vi "getAll.vi"(8 "error in (no error)":errorcluster, 11 "Instrument.sample-registry":refnum<class "Instrument.sample-registry.lvclass">) -> (0 "error out":errorcluster, 2 "getAll":variant, 3 "Instrument.sample-registry out":refnum<class "Instrument.sample-registry.lvclass">)   [LabVIEW 2019, in "Instrument.sample-registry.lvclass"]
uses:
  Instrument.sample-registry.lvclass
  Typedefs/Instrument.sample-registry.getAll--Cluster.ctl
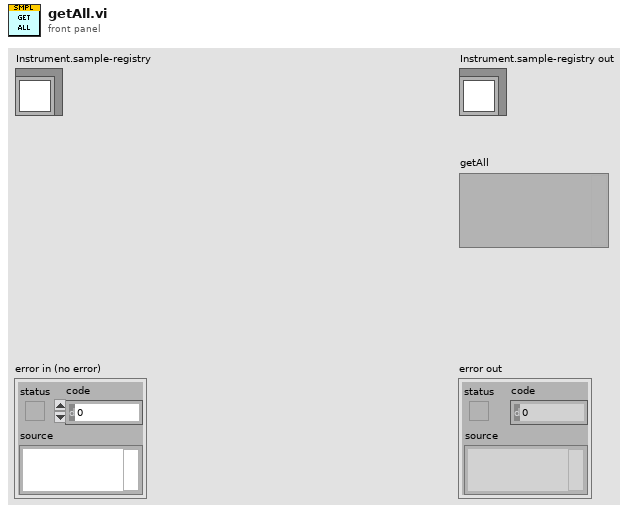
[diagram p1: front panel]
types:
  T1 = typedef "Instrument.sample-registry.lvclass/Instrument.sample-registry.getAll--Cluster.ctl" = cluster{"User":string, "Sample":string}
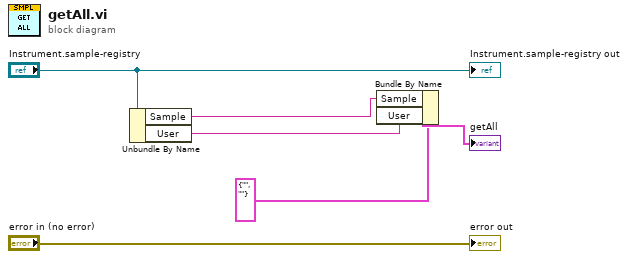
[diagram p0: block diagram]
diagram:
  n1 = Unbundle By Name("Instrument.sample-registry") -> ("Sample"=w2:string, "User"=w1:string)
  n2 = Bundle By Name(cluster=T1 {"User"="", "Sample"=""} ("getAll"), "Sample"=w2, "User"=w1) -> (→"getAll":T1)
  "error out" <- "error in (no error)"
  "Instrument.sample-registry out" <- "Instrument.sample-registry"
